vi "Terminate EtherNet_IP Connection.vi"(1 "error in":errorcluster, 2 "Connection Cluster":T1={"TCP Connection"=refnum, "Session"=[], "EtherNet/IP Device Address"="172.20.37.243"} {"Session" format="0x%02x"}) -> (0 "error out":errorcluster)   [LabVIEW 2020, in "EtherNet_IP_Lib.lvlib"]
uses:
  EtherNet_IP_Lib.lvlib
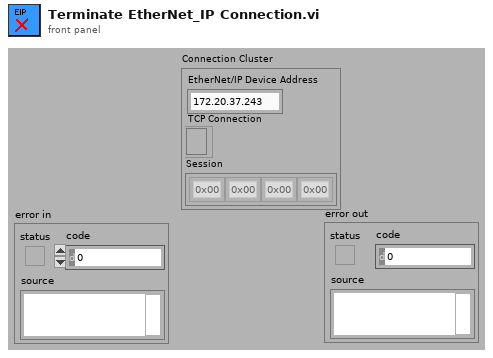
[diagram p1: front panel]
types:
  T1 = cluster{"TCP Connection":refnum<k5>, "Session":u8[], "EtherNet/IP Device Address":string}
  T2 = enum16{"Standard", "Buffered", "CRLF", "Immediate"}
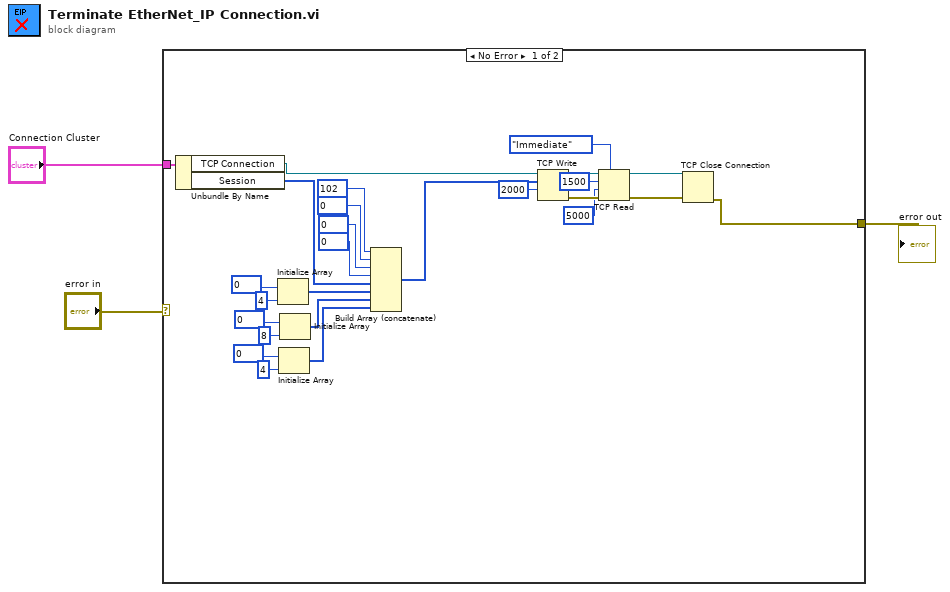
[diagram p0: block diagram]
diagram:
  n1 = case shown="No Error" "error in" {
    selector: "error in" -> [_ w30]
    tunnel: "Connection Cluster" -> [w13 _]
    tunnel: [w7 w30] -> w3
    frame No Error {
      n2 = Unbundle By Name(w13) -> ("TCP Connection"=w12:refnum<k5>, "Session"=w11:u8[])
      n3 = Initialize Array(u8 0 ("Status"), 4 ("dimension size")) -> (w27:u8[])
      n4 = Initialize Array(u8 0 ("Status"), 4 ("dimension size")) -> (w17:u8[])
      n5 = Initialize Array(u8 0 ("Status"), 8 ("dimension size")) -> (w18:u8[])
      n6 = Build Array (concatenate)(u8 102 ("Status"), u8 0 ("Status"), u8 0 ("Status"), u8 0 ("Status"), w11, w27, w18, w17) -> (w16:u8[])
      n7 = TCP Write(connection ID=w12, data in=w16, 9:2000 ("timeout ms (25000)")) -> (connection ID out=w14:refnum<k5>, error out=w15:errorcluster)  [unwired: 1 in, 1 out]
      n8 = TCP Read(connection ID=w14, bytes to read=1500, error in (no error)=w15, 7:T2."Immediate" ("mode (standard)"), 9:5000 ("timeout ms (25000)")) -> (connection ID out=w9:refnum<k5>, error out=w8:errorcluster)  [unwired: 1 out]
      n9 = TCP Close Connection(connection ID=w9, error in (no error)=w8) -> (error out=w7:errorcluster)  [unwired: 1 in, 1 out]
    }
    frame Error {
    }
  }
  "error out" <- w3
